vi "StartManageMenu.vi"(8 "error in (no error)":errorcluster, 11 "Menu in":refnum<class "Menu.lvclass">) -> (0 "error out":errorcluster, 3 "Menu out":refnum<class "Menu.lvclass">)   [LabVIEW 2021, in "Menu.lvlib" / "Menu.lvclass"]
uses:
  Menu.lvclass
  TR_ManageMenu.vi
  Menu.lvclass/Menu.ctl
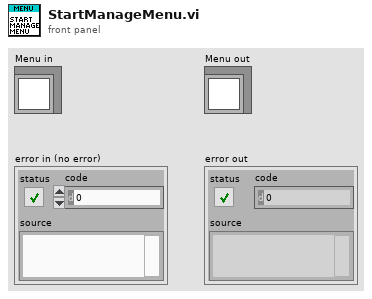
[diagram p1: front panel]
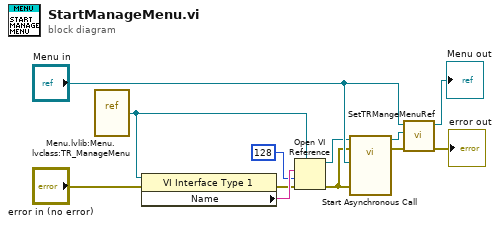
[diagram p0: block diagram]
diagram:
  n1 = vi-ref "Menu.lvlib:Menu.lvclass:TR_ManageMenu.vi"() -> (w2:refnum<vi>)
  n2 = property class="VI Interface Type 1"(reference=w2, error in="error in (no error)") -> (error out=w3:errorcluster, "Name"=w6:string)  [unwired: 1 out]
  n3 = Open VI Reference(type specifier VI Refnum (for type only)=w2, vi path=w6, options=128, error in (no error)=w3) -> (vi reference=w1:refnum<vi>, error out=w7:errorcluster)  [unwired: 2 in]
  n4 = call-by-ref "Start Asynchronous Call"(reference=w1, error in=w7, 8:"error in (no error)"=w7, "Menu in"="Menu in") -> (reference out=w12:refnum<vi>, error out=w8:errorcluster)  [unwired: 9 in, 1 out]
  n5 = call "SetTRMangeMenuRef.vi"("error in (no error)"=w8, "TR_ManageMenuRef"=w12, "Menu in"="Menu in") -> ("error out"=→"error out":errorcluster, "Menu out"=→"Menu out":refnum<class "Menu.lvclass">)  [unwired: 7 in]
